vi "Present Data.vi"(8 "error in (no error)":errorcluster, 10 "Debug Data":refnum<class "Debug Data.lvclass">[](array[class]), 11 "List Seen Processes View Model In":refnum<class "List Messages View Model.lvclass">) -> (0 "error out":errorcluster, 3 "List Seen Processes View Model Out":refnum<class "List Messages View Model.lvclass">)   [LabVIEW 2020, in "List Messages View Model.lvclass"]
uses:
  List Messages View Model.lvclass
  Debug Data/Debug Data.lvclass
  Debug Data/Debug Data.lvclass/Debug Data.ctl
panel:
  out "Message List":string[](array[string])
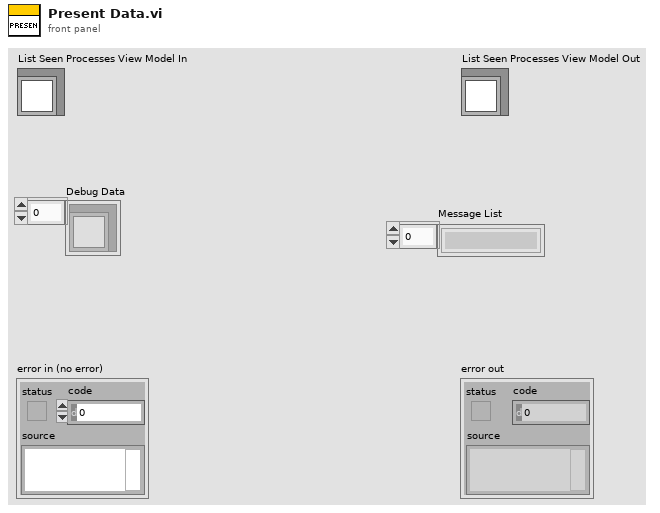
[diagram p1: front panel]
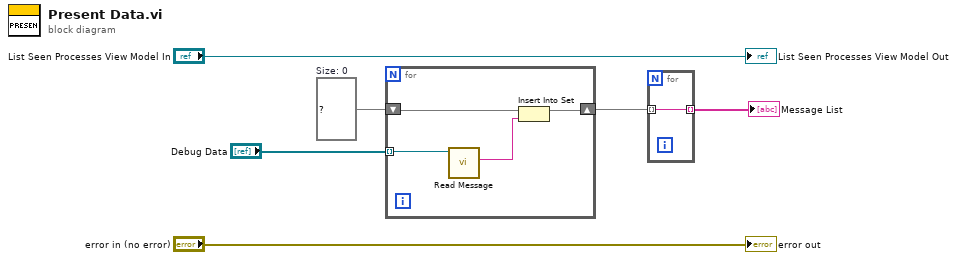
[diagram p0: block diagram]
diagram:
  w3 = set{string} {}  # Size: 0
  n1 = for {
    tunnel: "Debug Data" -> [w10] mode=indexing
    shift-right: [w7] -> w1
    shift-left: w3 -> [w9]
    n2 = call "Read Message.vi"("Debug Data in"=w10) -> ("Message"=w8:string)  [unwired: 7 in, 3 out]
    n3 = Insert Into Set(10:w8, 11:w9) -> (3:w7:set{string})  [unwired: 1 out]
  }
  n4 = for {
    tunnel: [w11] -> w2 mode=indexing
    tunnel: w1 -> [w11] mode=indexing
  }
  "Message List" <- w2
  "error out" <- "error in (no error)"
  "List Seen Processes View Model Out" <- "List Seen Processes View Model In"
